vi "Queue Init.vi"(8 "error in (no error)":errorcluster caption="Error In", 10 "Queue Name":string, 11 "Max":i32=-1) -> (0 "错误输出":errorcluster, 2 "New?":bool, 3 "Queue Out":refnum<queue>)   [LabVIEW 2020]
uses:
  Queue Message.ctl
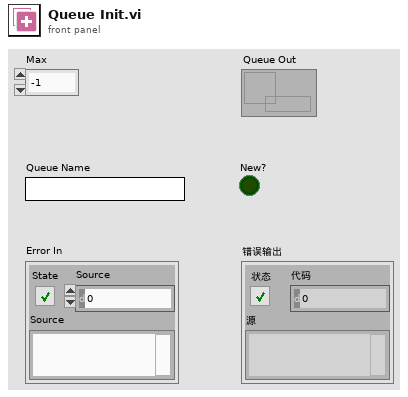
[diagram p1: front panel]
types:
  T1 = enum16{"Read Queue", "Add Queue", "Delete Queue"}
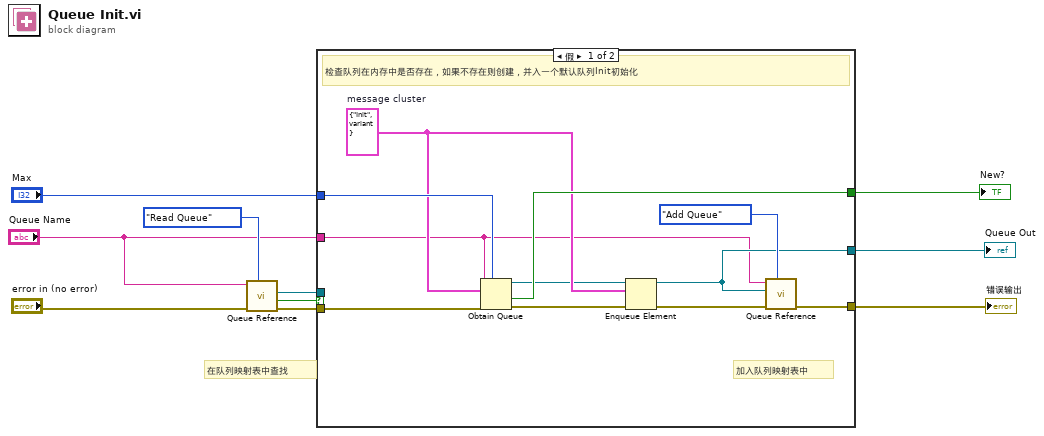
[diagram p0: block diagram]
diagram:
  # "在队列映射表中查找"
  n1 = call "Queue Reference.vi"("Mode"=T1."Read Queue", "Error In"="error in (no error)", "Name"="Queue Name") -> ("Error Out"=w4:errorcluster, "Found?"=w2:bool, "Queue Out"=w1:refnum<queue>)  [unwired: 5 in, 1 out]
  n2 = case shown="假" w2 {
    tunnel: "Max" -> [w21 _]
    tunnel: [w20 _] -> w9
    tunnel: [w14 w22] -> w8
    tunnel: [w13 w23] -> w7
    tunnel: w4 -> [w12 w22]
    tunnel: "Queue Name" -> [w11 _]
    tunnel: w1 -> [_ w23]
    frame False {
      w17 = cluster{"message":string, "data":variant} {"message"="Init", "data"=variant}  # message cluster
      # "加入队列映射表中"
      # "检查队列在内存中是否存在，如果不存在则创建，并入一个默认队列Init初始化"
      n3 = Obtain Queue(max queue size (-1, unlimited)=w21, name (unnamed)=w11, element data type=w17, error in (no error)=w12) -> (queue out=w16:refnum<queue>, created new?=w20:bool, error out=w18:errorcluster)  [unwired: 1 in]
      n4 = Enqueue Element(queue=w16, element=w17, error in (no error)=w18) -> (queue out=w13:refnum<queue>, error out=w15:errorcluster)  [unwired: 1 in, 1 out]
      n5 = call "Queue Reference.vi"("Mode"=T1."Add Queue", "Error In"=w15, "Queue In"=w13, "Name"=w11) -> ("Error Out"=w14:errorcluster)  [unwired: 4 in, 3 out]
    }
    frame True {
      # "检查队列在内存中是否存在，如果存在则直接根据名称从映射表中取出并使用"
    }
  }
  "New?" <- w9
  "Queue Out" <- w7
  "错误输出" <- w8
